vi "Catch.vi"   [LabVIEW 2015, in "LV Exceptions v1.lvlib"]
uses:
  LV Exceptions v1.lvlib
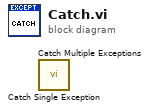
[diagram p0: block diagram]
diagram:
  n1 = call "Catch Single Exception.vi"() -> ()  [unwired: 13 in, 3 out]
  n2 = call "Catch Multiple Exceptions.vi"() -> ()  [unwired: 13 in, 3 out]
